vi "Triangle Wave PtByPt.vi"(1 "time":dbl format="%0.2f", 2 "phase":dbl format="%0.2f", 3 "frequency":dbl=1.0 format="%0.2f", 4 "amplitude":dbl=1.0 format="%0.2f") -> (0 "triangle wave":dbl format="%0.2f")   [LabVIEW 2017, in "NI_PtbyPt.lvlib"]
doc: "Generates a triangle wave point by point."
uses:
  <vilib>/ptbypt/NI_PtbyPt.lvlib
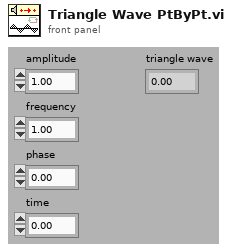
[diagram p1: front panel]
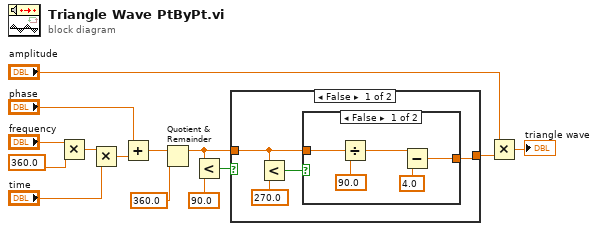
[diagram p0: block diagram]
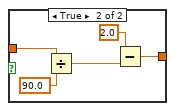
[diagram p2: hidden frame]
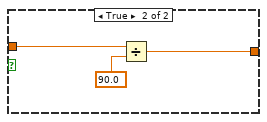
[diagram p3: hidden frame]
diagram:
  n1 = Multiply(x="frequency", y=360.0 ("x")) -> (x*y=w14:dbl)
  n2 = Multiply(x=w14, y="time") -> (x*y=w10:dbl)
  n3 = Add(x="phase", y=w10) -> (x+y=w9:dbl)
  n4 = Quotient & Remainder(x=w9, y=360.0) -> (x-y*floor(x/y)=w6:dbl)  [unwired: 1 out]
  n5 = Less?(x=w6, y=90.0) -> (x < y?=w7:bool)
  n6 = case shown="False" w7 {
    tunnel: w6 -> [w16 w31]
    tunnel: [w15 w29] -> w5
    frame False {
      n7 = Less?(x=w16, y=270.0) -> (x < y?=w17:bool)
      n8 = case shown="False" w17 {
        tunnel: w16 -> [w22 w27]
        tunnel: [w19 w24] -> w15
        frame False {
          n9 = Divide(x=w22, y=90.0) -> (x/y=w21:dbl)
          n10 = Subtract(x=w21, y=4.0) -> (x-y=w19:dbl)
        }
        frame True {
          n11 = Divide(x=w27, y=90.0) -> (x/y=w25:dbl)
          n12 = Subtract(x=2.0, y=w25) -> (x-y=w24:dbl)
        }
      }
    }
    frame True {
      n13 = Divide(x=w31, y=90.0) -> (x/y=w29:dbl)
    }
  }
  n14 = Multiply(x="amplitude", y=w5) -> (x*y=→"triangle wave":dbl)
